vi "Pre Launch Init.vi"(11 "Event Source In":refnum<class "Event Source.lvclass">) -> (0 "Error Out":errorcluster, 3 "Event Source Out":refnum<class "Event Source.lvclass">)   [LabVIEW 2019, in "Event Source.lvlib" / "Event Source.lvclass"]
doc: "(<B>Filename</B>: Actor Framework.lvlib:Actor.lvclass:Pre Launch Init.vi)\n\nDefines behavior that occurs after the Launch Nested Actor method is invoked but before the actor's Actor Core method begins running.\n\nBy default, this method does nothing. A descendant class may override it to define behavior."
uses:
  Event Source.lvclass
  <vilib>/ActorFramework/Actor/Actor.lvclass
  <vilib>/ActorFramework/Message Enqueuer/Message Enqueuer.lvclass
  Event Source Messages/Event Generated Msg/Event Generated Msg.lvclass
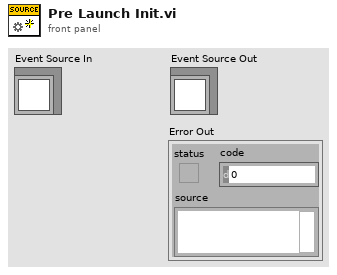
[diagram p1: front panel]
types:
  T1 = map{string, map{refnum<class "Message Enqueuer.lvclass">, refnum<class "Event Generated Msg.lvclass">}}
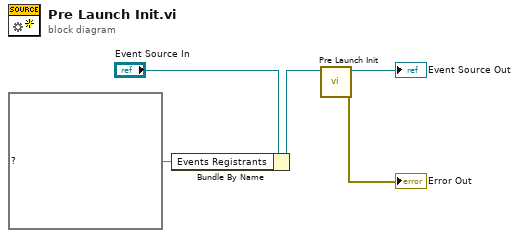
[diagram p0: block diagram]
diagram:
  n1 = Bundle By Name(cluster="Event Source In", "Events Registrants"=T1 {}) -> (w3:refnum<class "Event Source.lvclass">)
  n2 = call-parent "Pre Launch Init.vi"("Actor in"=w3) -> ("error out"=→"Error Out":errorcluster, "Actor out"=→"Event Source Out":refnum<class "Event Source.lvclass">)  [unwired: 9 in]
